vi "Apply General Configuration.vi"(7 "Restart (T)":bool=TRUE, 8 "error in (no error)":errorcluster, 9 "Cell Inhibit Enable":bool, 10 "Protocol (Legacy)":T1, 11 "Ethernet in":refnum<class "ENET_BS1201.lvclass">) -> (0 "error out":errorcluster, 3 "Ethernet out":refnum<class "ENET_BS1201.lvclass">)   [LabVIEW 2021, in "BS120x Driver.lvlib" / "ENET_BS1201.lvclass"]
doc: "DEPRECATED for BS1201 \nno general config anymore; BS1201 can handle ENET and CAN at the same time.\nENET has ability to disable broadcast"
uses:
  ENET_BS1201.lvclass
  TypeDefs/Protocol.ctl
  ENET_BS1201.lvclass/ENET_BS1201.ctl
  BS120x.lvclass
panel:
  # "no general config anymore; BS1201 can handle ENET and CAN at the same time.\nENET has ability to disable broadcast"
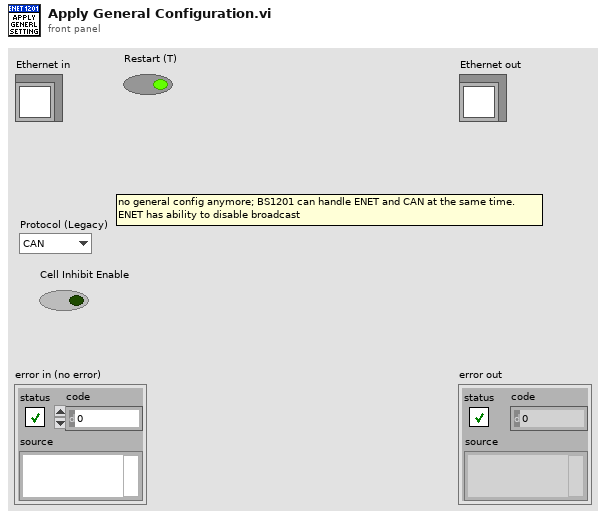
[diagram p1: front panel]
types:
  T1 = typedef "BS120x Driver.lvlib/BS120x.lvclass/Protocol.ctl" = enum16{"CAN", "Ethernet"}
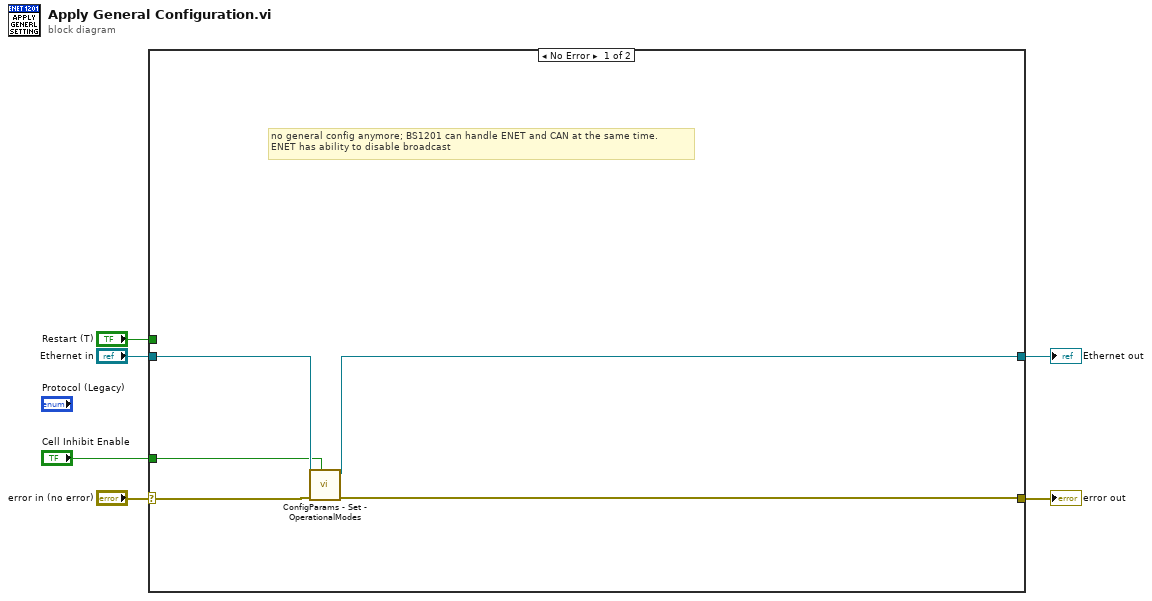
[diagram p0: block diagram]
diagram:
  n1 = case shown="No Error" "error in (no error)" {
    selector: "error in (no error)" -> [w11 w13]
    tunnel: [w7 w13] -> w5
    tunnel: [w9 w12] -> w3
    tunnel: "Ethernet in" -> [w10 w12]
    tunnel: "Restart (T)" -> [_ _]
    tunnel: "Cell Inhibit Enable" -> [w8 _]
    frame No Error {
      # "no general config anymore; BS1201 can handle ENET and CAN at the same time.\nENET has ability to disable broadcast"
      n2 = call-dynamic "ConfigParams - Set - OperationalModes.vi"("CellInhibitEnable"=w8, "error in (no error)"=w11, "Ethernet in"=w10) -> ("error out"=w7:errorcluster, "Ethernet out"=w9:refnum<class "ENET_BS1201.lvclass">)  [unwired: 7 in]
    }
    frame Error {
    }
  }
  "error out" <- w5
  "Ethernet out" <- w3
